vi "行列处理.vi"(1 "二维数组":dbl[][](array[numeric])) -> (0 "数组":dbl[][](array[numeric]))   [LabVIEW 2018]
uses:
  <vilib>/Analysis/baseanly.llb/Mean (DBL).vi
  <vilib>/Analysis/NI_AALBase.lvlib
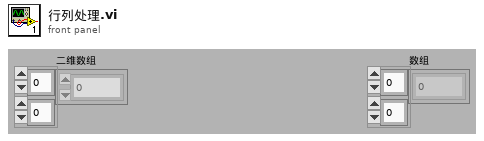
[diagram p1: front panel]
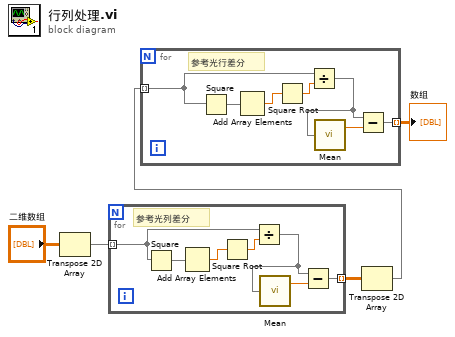
[diagram p0: block diagram]
diagram:
  n1 = Transpose 2D Array(2D array="二维数组") -> (transposed array=w4:dbl[][])
  n2 = for {
    tunnel: w4 -> [w6] mode=indexing
    tunnel: [w7] -> w5 mode=indexing
    # "参考光列差分"
    n3 = Square(x=w6) -> (x^2=w11:dbl[])
    n4 = Add Array Elements(numeric array=w11) -> (sum=w10:dbl)
    n5 = Square Root(x=w10) -> (sqrt(x)=w9:dbl)
    n6 = Divide(x=w6, y=w9) -> (x/y=w8:dbl[])
    n7 = call-poly <vilib>:"Mean.vi"("X"=w8) -> ("mean"=w12:dbl)  [unwired: 1 out]
    n8 = Subtract ("Subtract.vi")(x=w8, y=w12) -> (x-y=w7:dbl[])
  }
  n9 = Transpose 2D Array(2D array=w5) -> (transposed array=w3:dbl[][])
  n10 = for {
    tunnel: w3 -> [w15] mode=indexing
    tunnel: [w13] -> w1 mode=indexing
    # "参考光行差分"
    n11 = Square(x=w15) -> (x^2=w18:dbl[])
    n12 = Add Array Elements(numeric array=w18) -> (sum=w17:dbl)
    n13 = Square Root(x=w17) -> (sqrt(x)=w16:dbl)
    n14 = Divide(x=w15, y=w16) -> (x/y=w14:dbl[])
    n15 = call-poly <vilib>:"Mean.vi"("X"=w14) -> ("mean"=w19:dbl)  [unwired: 1 out]
    n16 = Subtract ("Subtract.vi")(x=w14, y=w19) -> (x-y=w13:dbl[])
  }
  "数组" <- w1
